vi "Progress bar galvanostatic calibration.vi"(2 "Range #":i32, 3 "Current (µA)":dbl format="%.3f", 4 "DAC code":u16) -> (0 "Abort":bool, 1 "Prog Bar Ref":refnum<vi>)   [LabVIEW 2015]
panel:
  in  "Abort":bool
  out "DAC code":u16(slide) scale=1000.0..12000.0
  # "Galvanostatic calibration progress"
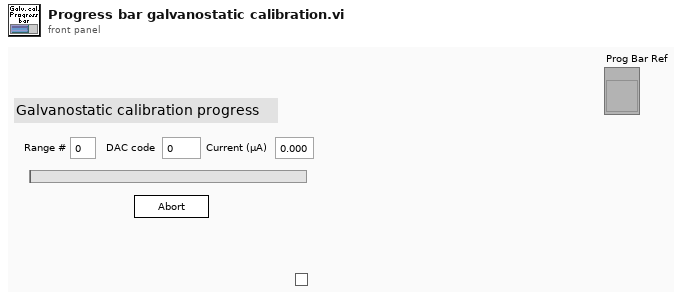
[diagram p1: front panel]
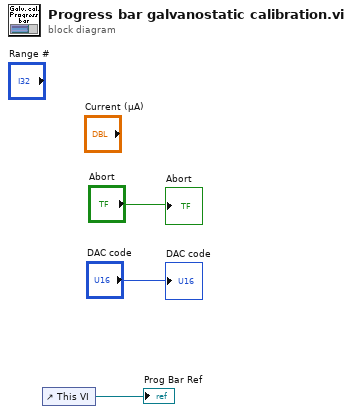
[diagram p0: block diagram]
diagram:
  n1 = control-ref of="This VI"() -> (→"Prog Bar Ref":refnum<vi>)
  "DAC code" <- "DAC code"
  "Abort" <- "Abort"
